vi "SV TDMS Write Order Level Components (NxM).vi"(0 "tdms file":refnum<k34>, 2 "write mode":u16(ring) items=["Append", "New group", "Overwrite"], 5 "group name in":string, 7 "channel names in":string[](array[string]), 9 "order components":cluster{"X":dbl[], "Y":dbl[]}[][](array[cluster]), 11 "error in":errorcluster, 12 "component":T1=32 items=["Magnitude"=32, "Phase"=33, "Real"=34, "Imaginary"=35, "Coherence"=36, "Unknown"=99], 13 "spectra info":T2[](array[typedef]) {"x-axis units" items=["Time (s)"=0, "Frequency-CB (Hz)"=1, "Frequency-CPB (Hz)"=1248, "Frequency-Arbitrary (Hz)"=2357, "Quefrency (s)"=2, "Revolutions (rev)"=3, "Order"=4, "Speed (RPM)"=11, "Speed (rad/s)"=21, "Index"=65535]; "weighting filter" items=["Linear", "A-weighting", "B-weighting", "C-weighting", "ITU-R 468-4", "Dolby", "CCITT", "C-message", "Wb", "Wc", "Wd", "We", "Wf", "Wh", "Wj", "Wk", "Wm", "AES17 20 kHz lowpass", "AES17 40 kHz lowpass", "AES17 20 kHz highpass", "AES17 40 kHz highpass"]; "dB reference [EU]" format="%.2f"; "engineering units" items=["custom..."=0, "V"=1, "A"=21, "C"=30, "pC"=31, "s"=32, "-"=29, "Pa"=2, "N"=20, "g"=3, "m/s^2"=4, "m/s"=5, "m"=6, "mm/s"=12, "mm"=13, "micron/s"=14, "micron"=15, "in/s^2"=7, "in/s"=8, "in"=9, "mil/s"=10, "mil"=11, "rad/s^2"=16, "rad/s"=17, "rad"=18, "deg/s^2"=26, "deg/s"=27, "deg"=28, "RPM"=22, "cycle/s^2"=23, "Hz"=24, "cycle"=25, "strain"=19]; "spectral info"."window" items=["None "=0, "Hanning"=1, "Hamming"=2, "Blackman-Harris"=3, "Exact Blackman"=4, "Blackman"=5, "Flat Top"=6, "4 Term B-Harris "=7, "7 Term B-Harris"=8, "Low Sidelobe"=9, "Force - Exponential"=10, "Gaussian"=62]}) -> (4 "tdms file out":refnum<k34>, 6 "group name out":string, 8 "channel names out":string[](array[string]), 15 "error out":errorcluster)   [LabVIEW 2017]
doc: "Writes data to the specified .tdms file in a format specific to the polymorphic instance. Wire data to the <B>scaled signal [EU]</B> input to determine the polymorphic instance to use or manually select the instance."
uses:
  <vilib>/addons/_NISVFA/_Shared subVIs/Controls/svc_Spectrum Info.ctl
  <vilib>/addons/_NISVFA/_Shared subVIs/Controls/svc_X-Axis Units.ctl
  <vilib>/addons/_NISVFA/_Shared subVIs/Controls/svc_Spectrum Type.ctl
  <vilib>/addons/_NISVFA/_Shared subVIs/Controls/svc_Engineering Units Text Ring.ctl
  <vilib>/addons/_NISVFA/_Shared subVIs/Controls/svc_Weighting Filter Text Ring.ctl
  <vilib>/addons/_NISVFA/_Shared subVIs/Controls/svc_Complimentary Spectrum Units.ctl
  <vilib>/addons/_NISVFA/_Shared subVIs/Controls/NI Spectrum Component.ctl
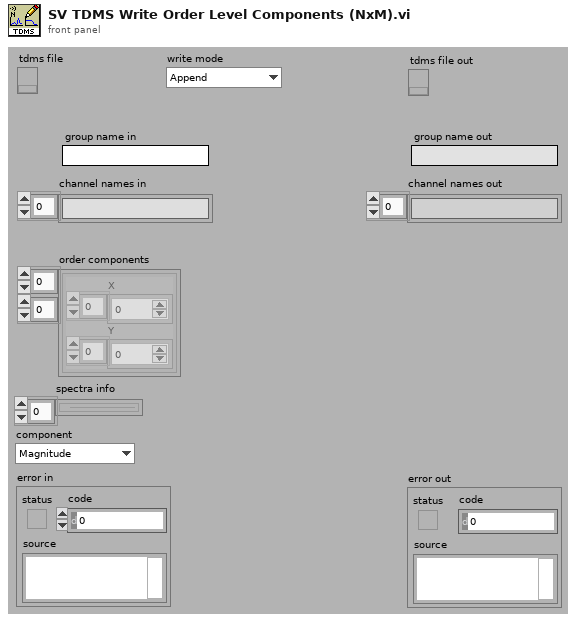
[diagram p1: front panel]
types:
  T1 = typedef "NI Spectrum Component.ctl" = u16
  T2 = typedef "svc_Spectrum Info.ctl" = cluster{"channel name":string, "description":string, "x-axis units":T3, "spectral info":cluster{"spectrum type":T4, "linear/dB":enum16{"linear", "dB"}, "window":u16, "window size":i32, "FFT size":i32}, "engineering units":T5, "custom label":string, "dB reference [EU]":dbl, "peak units":enum16{"rms", "peak", "peak-peak"}, "weighting filter":T6, "spectral density?":bool, "unit label":string, "spectrum skewed?":bool, "complimentary spectrum units":T7}
  T3 = typedef "svc_X-Axis Units.ctl" = u16
  T4 = typedef "svc_Spectrum Type.ctl" = enum16{"FFT Spectrum [complex]", "Amplitude [Magnitude]", "Power [Magnitude^2]", "Cross Spectrum [complex]", "Frequency Response [Complex]"}
  T5 = typedef "svc_Engineering Units Text Ring.ctl" = u16
  T6 = typedef "svc_Weighting Filter Text Ring.ctl" = u16
  T7 = typedef "svc_Complimentary Spectrum Units.ctl" = enum16{"none", "radians", "degrees", "cycles", "imaginary"}
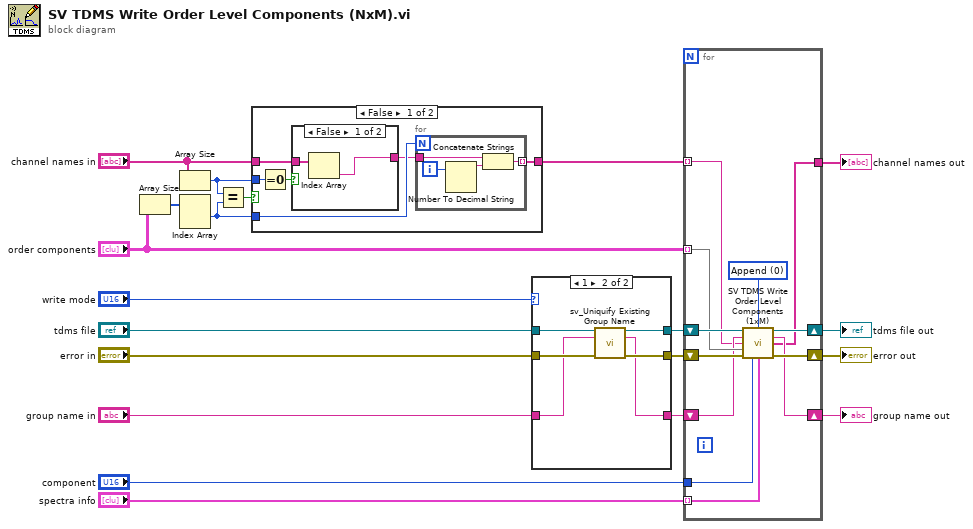
[diagram p0: block diagram]
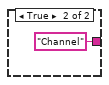
[diagram p3: hidden frame]
diagram:
  n1 = Array Size(array="order components") -> (size(s)=w14:i32[])
  n2 = Array Size(array="channel names in") -> (size(s)=w15:i32)
  n3 = Index Array(array=w14) -> (element #1=w12:i32)  [unwired: 2 in, 1 out]
  n4 = Equal?(x=w15, y=w12) -> (x = y?=w16:bool)
  n5 = case shown="False" w16 {
    tunnel: "channel names in" -> [w24 w34]
    tunnel: [w21 w34] -> w10
    tunnel: w15 -> [w26 _]
    tunnel: w12 -> [w23 _]
    frame False {
      n6 = Equal To 0?(x=w26) -> (x = 0?=w25:bool)
      n7 = case shown="False" w25 {
        tunnel: w24 -> [w32 _]
        tunnel: [w31 "Channel" ("channel name")] -> w22
        frame False {
          n8 = Index Array(array=w32) -> (element=w31:string)  [unwired: 1 in]
        }
        frame True {
        }
      }
      n9 = for {
        N: w23 -> [_]
        tunnel: w22 -> [w28]
        tunnel: [w27] -> w21 mode=indexing
        i -> [w29]
        n10 = Number To Decimal String(number=w29) -> (decimal integer string=w30:string)  [unwired: 1 in]
        n11 = Concatenate Strings(w28, w30) -> (w27:string)
      }
    }
    frame True {
    }
  }
  n12 = case shown="1" "write mode" {
    tunnel: [w37 w42] -> w8
    tunnel: [w35 w38] -> w4
    tunnel: "group name in" -> [w35 w39]
    tunnel: [w36 w40] -> w6
    tunnel: "error in" -> [w36 w41]
    tunnel: "tdms file" -> [w37 w43]
    frame 0, Default {
    }
    frame 1 {
      n13 = call <vilib>:"sv_Uniquify Existing Group Name.vi"("tdms file ref"=w43, "group name"=w39, "error in"=w41) -> ("tdms file out"=w42:refnum<k34>, "unique group"=w38:string, "error out"=w40:errorcluster)  [unwired: 10 in]
    }
  }
  n14 = for {
    shift-right: [w51] -> w3
    shift-left: w8 -> [w55]
    shift-right: [w52] -> w2
    shift-left: w6 -> [w53]
    tunnel: "order components" -> [w54] mode=indexing
    tunnel: "spectra info" -> [w46] mode=indexing
    tunnel: "component" -> [w45]
    tunnel: [w48] -> w17
    tunnel: w10 -> [w47] mode=indexing
    shift-right: [w49] -> w18
    shift-left: w4 -> [w50]
    w44 = u16 0 items=["Append", "New group", "Overwrite"] ("write mode")
    n15 = call <vilib>:"SV TDMS Write Order Level Components (1xM).vi"("tdms file"=w55, "write mode"=w44, "group name in"=w50, "channel name in"=w47, "order component"=w54, "error in"=w53, "component"=w45, "spectrum info"=w46) -> ("tdms file out"=w51:refnum<k34>, "group name out"=w49:string, "channel names out"=w48:string[], "error out"=w52:errorcluster)  [unwired: 4 in]
  }
  "error out" <- w2
  "tdms file out" <- w3
  "group name out" <- w18
  "channel names out" <- w17
